vi "开发环境与运行环境的路径区别.vi"() -> ()   [LabVIEW 2017]
panel:
  out "stripped path 2":path
  out "stripped path":path
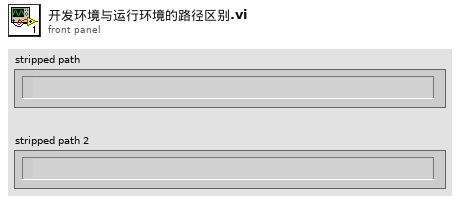
[diagram p1: front panel]
types:
  T1 = enum32{"invalid app kind", "Development System", "Run Time System", "Student Edition", "Embedded LabVIEW", "Evaluation", "Custom"}
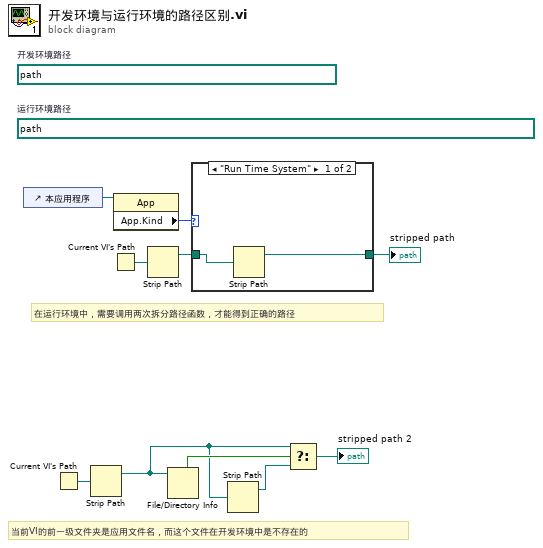
[diagram p0: block diagram]
diagram:
  (unwired) path "C:/Users/vs/Desktop/开放环境与运行环境的路径区别.EXE/开放环境与运行环境的路径区别.vi"  # 运行环境路径
  (unwired) path "C:/Users/vs/Desktop/开放环境与运行环境的路径区别.vi"  # 开发环境路径
  # "当前VI的前一级文件夹是应用文件名，而这个文件在开发环境中是不存在的"
  # "在运行环境中，需要调用两次拆分路径函数，才能得到正确的路径"
  n1 = control-ref of="本应用程序"() -> (w10:refnum<vi>)
  n2 = Current VI's Path() -> (path=w8:path)
  n3 = Strip Path(path=w8) -> (stripped path=w6:path)  [unwired: 1 out]
  n4 = Current VI's Path() -> (path=w9:path)
  n5 = property class="App"(reference=w10) -> ("App.Kind"=w3:T1)  [unwired: 1 in, 2 out]
  n6 = Strip Path(path=w9) -> (stripped path=w2:path)  [unwired: 1 out]
  n7 = File/Directory Info(path=w6) -> (directory=w7:bool)  [unwired: 1 in, 6 out]
  n8 = case shown="\"Run Time System\"" w3 {
    tunnel: w2 -> [w12 w13]
    tunnel: [w11 w13] -> w1
    frame "Run Time System" {
      n9 = Strip Path(path=w12) -> (stripped path=w11:path)  [unwired: 1 out]
    }
    frame "Development System", Default {
    }
  }
  "stripped path" <- w1
  n10 = Strip Path(path=w6) -> (stripped path=w5:path)  [unwired: 1 out]
  n11 = Select(t=w6, s=w7, f=w5) -> (s? t:f=→"stripped path 2":path)
